vi "Match Elevator Position and Location.vi"(8 "error in (no error)":errorcluster, 10 "Elevator Position":T1, 11 "Elevator Controller Actor in":refnum<class "Elevator Controller Actor.lvclass">) -> (0 "error out":errorcluster, 3 "Elevator Controller Actor out":refnum<class "Elevator Controller Actor.lvclass">)   [LabVIEW 2019, in "Elevator Controller Actor.lvlib" / "Elevator Controller Actor.lvclass"]
uses:
  Elevator Controller Actor.lvclass
  Simulated Sensor Interface Actor/Sim Sensor Interface Messages/Write Elevator Position Msg/Write Elevator Position Msg.lvclass
  Sim Display Console Actor/Elevator Controller/Floor -Enum.ctl
  Sim Display Console Actor/Elevator Controller/Sim Display Console Actor.lvclass
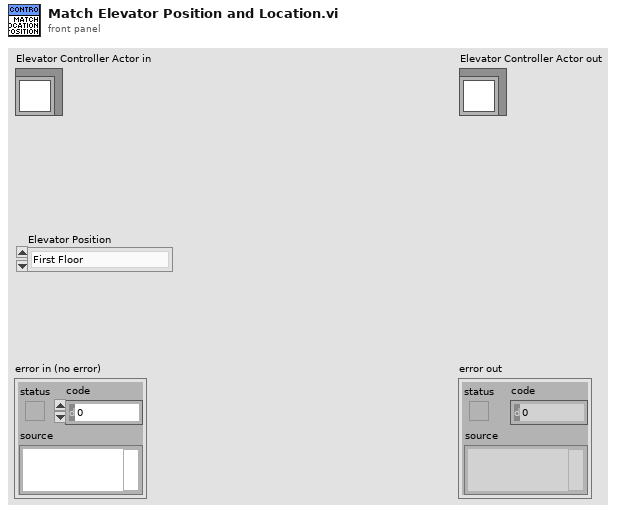
[diagram p1: front panel]
types:
  T1 = typedef "Simulated Display Console Actor.lvlib/Sim Display Console Actor.lvclass/Floor -Enum.ctl" = enum16{"First Floor", "Send Floor", "Third Floor", "Fourth Floor"}
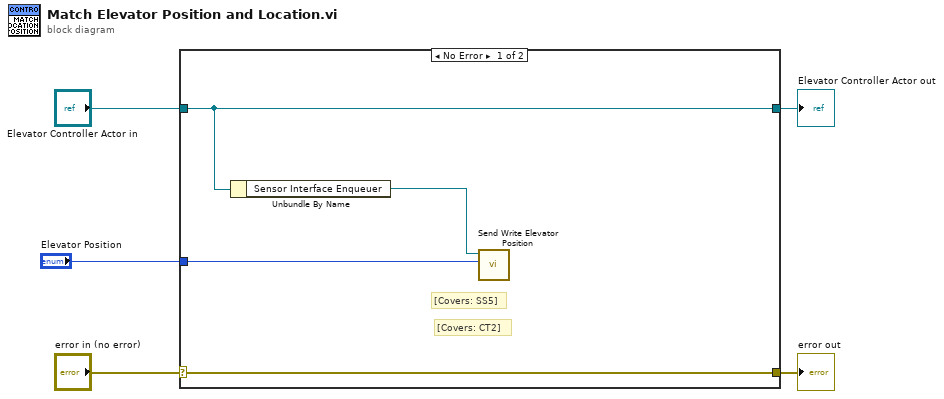
[diagram p0: block diagram]
diagram:
  n1 = case shown="No Error" "error in (no error)" {
    selector: "error in (no error)" -> [w9 w11]
    tunnel: [w9 w11] -> w4
    tunnel: [w8 w10] -> w2
    tunnel: "Elevator Controller Actor in" -> [w8 w10]
    tunnel: "Elevator Position" -> [w6 _]
    frame No Error {
      # "[Covers: CT2]"
      # "[Covers: SS5]"
      n2 = Unbundle By Name(w8) -> ("Sensor Interface Enqueuer"=w7:refnum<class "Message Enqueuer.lvclass">)
      n3 = call "Send Write Elevator Position.vi"("Elevator Position"=w6, "Message Enqueuer"=w7) -> ()  [unwired: 8 in, 2 out]
    }
    frame Error {
    }
  }
  "error out" <- w4
  "Elevator Controller Actor out" <- w2
